vi "Read Cell Type.vi"(8 "error in (no error)":errorcluster, 11 "Schedule Cell in":refnum<class "Schedule Cell.lvclass">) -> (0 "error out":errorcluster, 2 "Cell Type":string, 3 "Schedule Cell out":refnum<class "Schedule Cell.lvclass">)   [LabVIEW 2020, in "TALOS.lvlib" / "Run Utilities.lvlib" / "Schedule Cell.lvclass"]
uses:
  Schedule Cell.lvclass
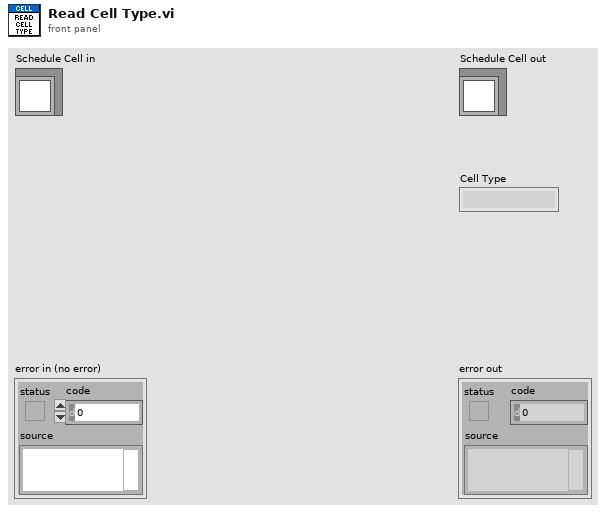
[diagram p1: front panel]
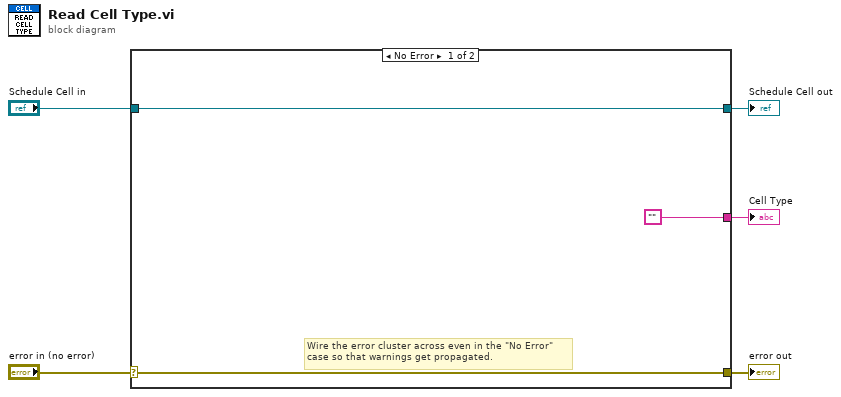
[diagram p0: block diagram]
diagram:
  n1 = case shown="No Error" "error in (no error)" {
    selector: "error in (no error)" -> [w7 w10]
    tunnel: [w7 w10] -> w4
    tunnel: [w8 w9] -> w2
    tunnel: "Schedule Cell in" -> [w8 w9]
    tunnel: ["" _] -> w1
    frame No Error {
      # "Wire the error cluster across even in the \"No Error\"\ncase so that warnings get propagated."
    }
    frame Error {
    }
  }
  "error out" <- w4
  "Schedule Cell out" <- w2
  "Cell Type" <- w1
